vi "Transcriptor LabVIEW to C code Step 4 Assign Output Values.vi"(8 "error in (no error)":errorcluster, 11 "Diagram in":refnum<vi>) -> (3 "output value assignement":string)   [LabVIEW 2014]
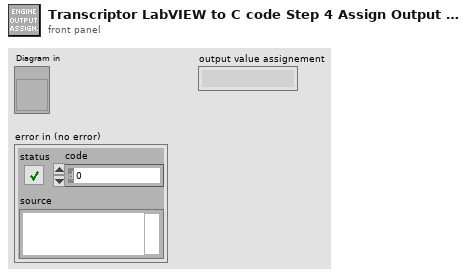
[diagram p1: front panel]
types:
  T1 = cluster{"wire labels":string[], "wire terminals datatypes":string[][]}
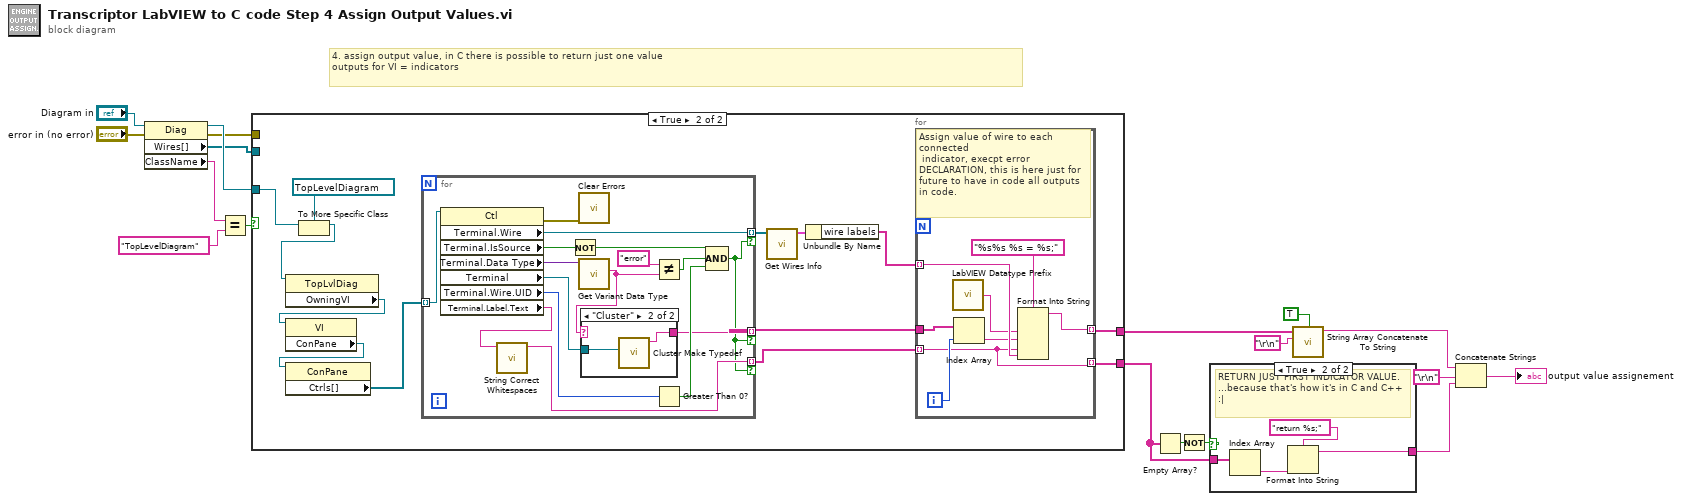
[diagram p0: block diagram]
diagram:
  # "4. assign output value, in C there is possible to return just one value\noutputs for VI = indicators"
  n1 = property class="Diag"(reference="Diagram in", error in="error in (no error)") -> (reference out=w17:refnum<vi>, error out=w2:errorcluster, "Wires[]"=w1:refnum<vi>[], "ClassName"=w18:string)
  n2 = Equal?(x=w18, y="TopLevelDiagram" ("Parent ClassName")) -> (x = y?=w15:bool)
  n3 = case shown="True" w15 {
    tunnel: w1 -> [_ _]
    tunnel: w2 -> [_ _]
    tunnel: [_ w31] -> w6
    tunnel: [_ w30] -> w11
    tunnel: w17 -> [_ w28]
    frame False {
    }
    frame True {
      n4 = To More Specific Class(target class=refnum<vi> refnum, reference=w28) -> (specific class reference=w27:refnum<vi>)  [unwired: 1 in, 1 out]
      n5 = property class="TopLvlDiag"(reference=w27) -> ("OwningVI"=w26:refnum<vi>)  [unwired: 1 in, 2 out]
      n6 = property class="VI"(reference=w26) -> ("ConPane"=w25:refnum<vi>)  [unwired: 1 in, 2 out]
      n7 = property class="ConPane"(reference=w25) -> ("Ctrls[]"=w24:refnum<vi>[])  [unwired: 1 in, 2 out]
      n8 = for {
        tunnel: w24 -> [w47] mode=indexing
        tunnel: [w34] -> w23 mode=indexing if=w32
        tunnel: [w36] -> w22 mode=indexing if=w32
        tunnel: [w33] -> w21 mode=indexing if=w32
        n9 = property class="Ctl"(reference=w47) -> (error out=w46:errorcluster, "Terminal.Wire"=w33:refnum<vi>, "Terminal.IsSource"=w45:bool, "Terminal.Data Type"=w44:variant, "Terminal"=w41:refnum<vi>, "Terminal.Wire.UID"=w40:i32, "Terminal.Label.Text"=w35:string)  [unwired: 1 in, 1 out]
        n10 = call "String Correct Whitespaces.vi"("String in"=w35) -> ("String out"=w34:string)  [unwired: 10 in]
        n11 = Not(x=w45) -> (.not. x?=w39:bool)
        n12 = call <vilib>:"Clear Errors.vi"("error in (no error)"=w46) -> ()  [unwired: 5 in, 2 out]
        n13 = call "Get Variant Data Type.vi"("Variant in"=w44) -> ("first data type"=w42:string)  [unwired: 9 in, 1 out]
        n14 = case shown="\"Cluster\"" w42 {
          selector: w42 -> [w48 _]
          tunnel: [w48 w50] -> w36
          tunnel: w41 -> [_ w49]
          frame Default {
          }
          frame "Cluster" {
            n15 = call "Cluster Make Typedef.vi"("Terminal in"=w49) -> ("typedfinition"=w50:string)  [unwired: 8 in, 2 out]
          }
        }
        n16 = Not Equal?(x="error", y=w42) -> (x != y?=w38:bool)
        n17 = Greater Than 0?(x=w40) -> (x > 0?=w37:bool)
        n18 = Compound Arithmetic op=AND(w39, w38, w37) -> (w32:bool)
      }
      n19 = call "Get Wires Info.vi"("connected\nwires refs."=w21) -> ("wires info cluster"=w20:T1)  [unwired: 10 in]
      n20 = Unbundle By Name(w20) -> ("wire labels"=w19:string[])
      n21 = for {
        tunnel: w23 -> [w51] mode=indexing
        tunnel: w19 -> [w56] mode=indexing
        tunnel: [w57] -> w31 mode=indexing
        tunnel: w22 -> [w54]
        tunnel: [w51] -> w30 mode=indexing
        i -> [w55]
        # "Assign value of wire to each connected\n indicator, execpt error\nDECLARATION, this is here just for future to have in code all outputs in code."
        n22 = call "LabVIEW Datatype Prefix.vi"() -> ("datatype prefix"=w52:string)
        n23 = Index Array(array=w54, index=w55) -> (element=w53:string)
        n24 = Format Into String(format string="%s%s %s = %s;", w52, w53, w51, w56) -> (resulting string=w57:string)  [unwired: 2 in, 1 out]
      }
    }
  }
  n25 = Empty Array?(array=w11) -> (empty?=w12:bool)
  n26 = Not(x=w12) -> (.not. x?=w13:bool)
  n27 = case shown="True" w13 {
    tunnel: [_ w60] -> w9
    tunnel: w11 -> [_ w59]
    frame False {
    }
    frame True {
      # "RETURN JUST FIRST INDICATOR VALUE.\n...because that's how it's in C and C++ :|"
      n28 = Index Array(array=w59) -> (element=w61:string)  [unwired: 1 in]
      n29 = Format Into String(format string="return %s;", w61) -> (resulting string=w60:string)  [unwired: 2 in, 1 out]
    }
  }
  n30 = call "String Array Concatenate To String.vi"("insert last delimiter?"=TRUE, "Delimiter char"="\r\n", "Array String In"=w6) -> ("String"=w8:string)  [unwired: 8 in]
  n31 = Concatenate Strings(w8, "\r\n", w9) -> (→"output value assignement":string)
